vi "Test1.vi"() -> ()   [LabVIEW 2019, in "Inst.MOTOR.lvclass"]
uses:
  Inst.MOTOR.lvclass
  Typedefs/Inst.MOTOR.Configuration--Cluster.ctl
  Inst.MOTOR.lvclass/Inst.MOTOR.ctl
  <vilib>/addons/_JKI Toolkits/Caraya/classes/Assert/Assert Not Error.vi
  <vilib>/addons/_JKI Toolkits/Caraya/classes/Assert/Assert.lvclass
  <vilib>/addons/_JKI Toolkits/Caraya/classes/Test/Test.lvclass
panel:
  out "read buffer":string
  in  "write buffer":string
  in  "Configuration":T1={"baud rate"=9600, "data bits"=8, "parity"=enum."None", "stop bits"=10, "flow control"=0, "Read Count"=1000, "Address"="", "Termination Character"=10} {"Termination Character" format="%.0x"; "flow control" items=["None"=0, "XON/XOFF"=1, "RTS/CTS"=2, "DTR/DSR"=4]; "stop bits" items=["1.0"=10, "1.5"=15, "2.0"=20]; "data bits" min=5 max=8 step=1; "baud rate" items=["75"=75, "110"=110, "134"=134, "150"=150, "300"=300, "600"=600, "1200"=1200, "1800"=1800, "2400"=2400, "4800"=4800, "7200"=7200, "9600"=9600, "14400"=14400, "19200"=19200, "28800"=28800, "38400"=38400, "56000"=56000, "57600"=57600, "115200"=115200, "128000"=128000, "230400"=230400]}
  out "error out":errorcluster
  # "0xA is equivalent to a '\\n' character, which is a line feed."
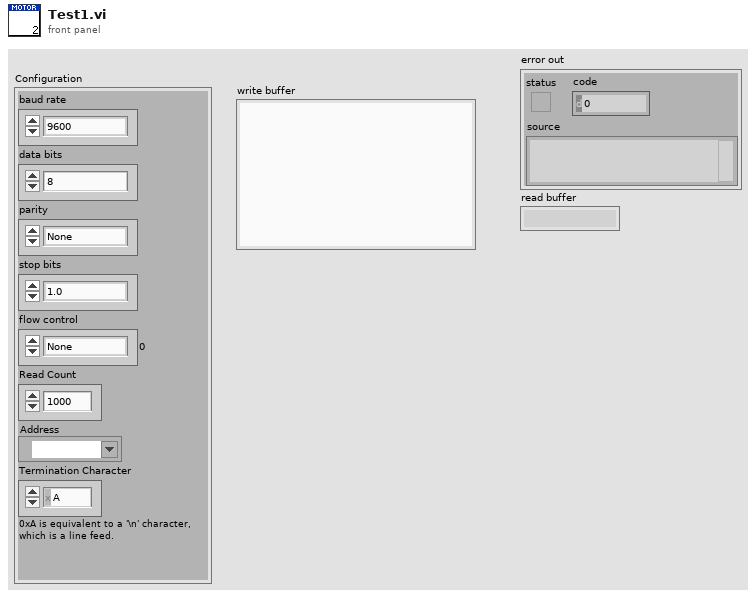
[diagram p1: front panel]
types:
  T1 = typedef "Inst.MOTOR.lvclass/Inst.MOTOR.Configuration--Cluster.ctl" = cluster{"baud rate":u32, "data bits":u16, "parity":enum16{"None", "Odd", "Even", "Mark", "Space"}, "stop bits":u16, "flow control":u16, "Read Count":u32, "Address":refnum<visa-resource-name>, "Termination Character":u8}
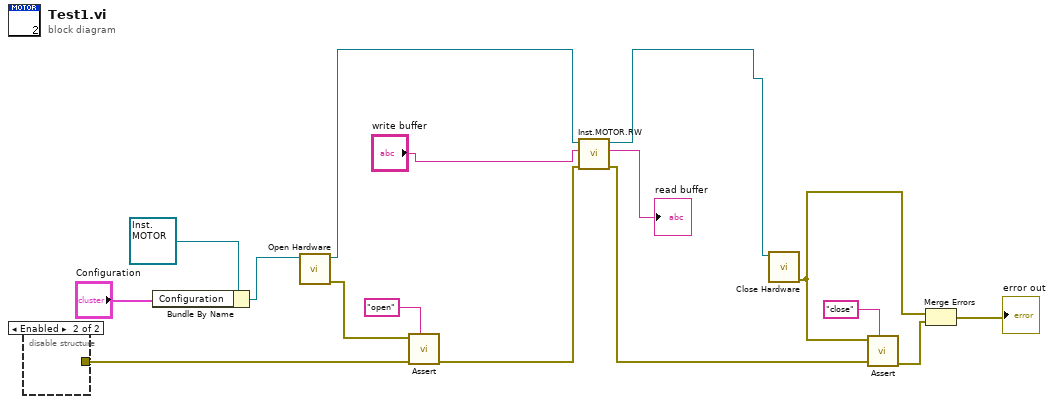
[diagram p0: block diagram]
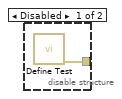
[diagram p2: hidden frame]
diagram:
  n1 = disable-structure shown="Enabled" {
    disable-tunnel: [w17 _] -> w8
    frame Disabled {
      n2 = call <vilib>:"Define Test.vi"() -> ("error out"=w17:errorcluster)  [unwired: 10 in, 1 out]
    }
    frame Enabled {
    }
  }
  n3 = Bundle By Name(cluster=refnum<class "Inst.MOTOR.lvclass"> refnum ("Inst.MOTOR in"), "Configuration"="Configuration") -> (w15:refnum<class "Inst.MOTOR.lvclass">)
  n4 = call-dynamic "Open Hardware.vi"("Inst.MOTOR in"=w15) -> ("error out"=w7:errorcluster, "Inst.MOTOR out"=w6:refnum<class "Inst.MOTOR.lvclass">)  [unwired: 9 in]
  n5 = call-poly <vilib>:"Assert.vi"("Label"="open", "error in (no error)"=w8, "Not Error?"=w7) -> ("error out"=w3:errorcluster)  [unwired: 7 in, 1 out]
  n6 = call "Inst.MOTOR.RW.vi"("error in (no error)"=w3, "Data in"="write buffer", "Inst.MOTOR in"=w6) -> ("error out"=w2:errorcluster, "read buffer"=→"read buffer":string, "Inst.MOTOR out"=w1:refnum<class "Inst.MOTOR.lvclass">)  [unwired: 6 in]
  n7 = call-dynamic "Close Hardware.vi"("Inst.MOTOR in"=w1) -> ("error out"=w10:errorcluster)  [unwired: 9 in, 1 out]
  n8 = call-poly <vilib>:"Assert.vi"("Label"="close", "error in (no error)"=w2, "Not Error?"=w10) -> ("error out"=w11:errorcluster)  [unwired: 7 in, 1 out]
  n9 = Merge Errors(w10, w11) -> (→"error out":errorcluster)
